vi "PONG.vi"(6 "timeout ms (conn default)":i32=-2, 8 "error in":errorcluster, 11 "nats connection in":T1={"connection ID"=refnum, "server INFO"="", "timeout ms"=5000, "verbose?"=FALSE, "server headers?"=FALSE, "client headers?"=FALSE}) -> (0 "error out":errorcluster, 3 "dup nats connection":T1={"connection ID"=refnum, "server INFO"="", "timeout ms"=5000, "verbose?"=FALSE, "server headers?"=FALSE, "client headers?"=FALSE})   [LabVIEW 2013, in "NATS Core.lvlib"]
doc: "Sends a PONG response to the NATS server."
uses:
  NATS Core.lvlib
  Controls/nats connection.ctl
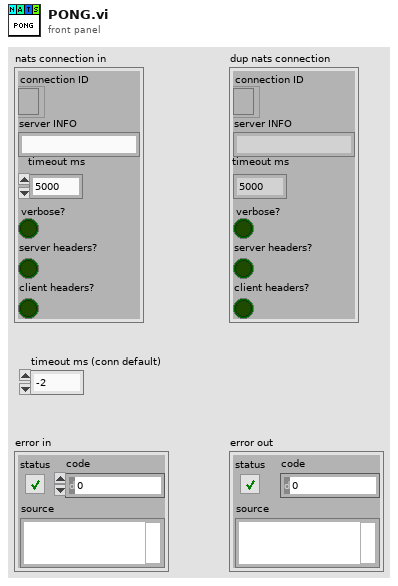
[diagram p1: front panel]
types:
  T1 = typedef "NATS Core.lvlib/nats connection.ctl" = cluster{"connection ID":refnum<k5>, "server INFO":string, "timeout ms":i32, "verbose?":bool, "server headers?":bool, "client headers?":bool}
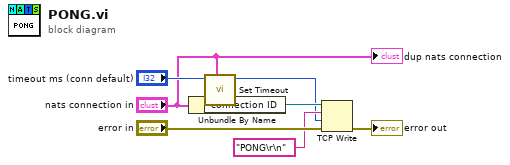
[diagram p0: block diagram]
diagram:
  n1 = Unbundle By Name("nats connection in") -> ("connection ID"=w6:refnum<k5>)
  n2 = call "Set Timeout.vi"("nats connection in"="nats connection in", "timeout ms in"="timeout ms (conn default)") -> ("timeout ms out"=w1:i32)  [unwired: 9 in]
  n3 = TCP Write(connection ID=w6, data in="PONG\r\n", error in (no error)="error in", 9:w1) -> (error out=→"error out":errorcluster)  [unwired: 2 out]
  "dup nats connection" <- "nats connection in"
